vi "Update Humidity Control.vi"(8 "error in":errorcluster, 11 "cCRDS in":refnum<class "cCRDS.lvclass">=refnum) -> (0 "error out":errorcluster, 3 "cCRDS out":refnum<class "cCRDS.lvclass">)   [LabVIEW 2015, in "cCRDS.lvclass"]
uses:
  cCRDS.lvclass
  cCRDS.lvclass/cCRDS.ctl
  Reusable/CRDS/Cell/CRDS Cell.lvclass/CRDS Cell.ctl
  <vilib>/DAQmx/write.llb/DAQmx Write (Analog 1D DBL NChan 1Samp).vi
  Reusable/CRDS/Cell/Read Data.vi
  <vilib>/DAQmx/miscellaneous.llb/DAQmx Fill In Error Info.vi
  Reusable/CRDS/Main/Read Cells.vi
  Reusable/CRDS/Data/Cell/Read hkParam.vi
  Reusable/Humidity Control/Multi-Loop Humidity Control.vi
  Reusable/CRDS/Cell/CRDS Cell.lvclass
  Reusable/CRDS/Data/Cell/CRDS Cell Data.lvclass
  Reusable/General/Temperature/Temperature.lvlib
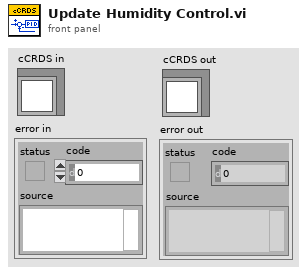
[diagram p1: front panel]
types:
  T1 = cluster{"Array of Single[0]":sgl, "Array of Single[1]":sgl, "Array of Single[2]":sgl}
  T2 = cluster{"Array of Single[0]":sgl, "Array of Single[1]":sgl, "Array of Single[2]":sgl}[]
  T3 = typedef "calData.ctl" = cluster{"rhDilFac":sgl, "Q":sgl, "Tmean":sgl, "extDilFac":sgl, "rhCell":sgl, "P":sgl, "T":sgl}
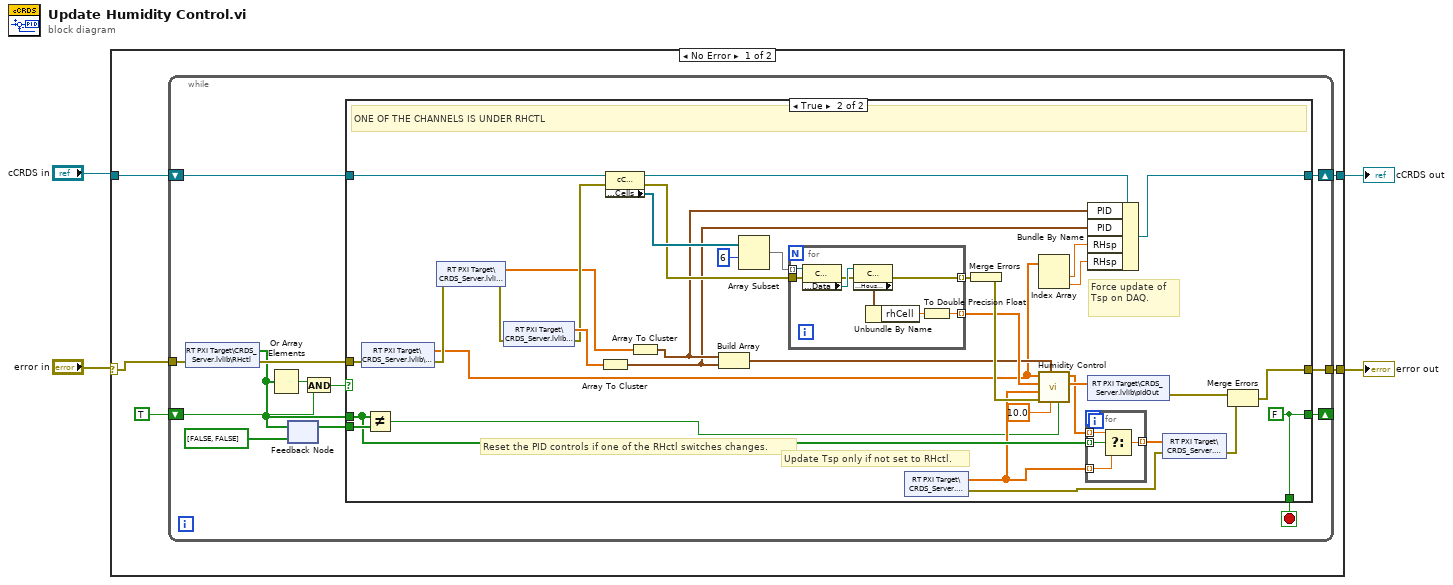
[diagram p0: block diagram]
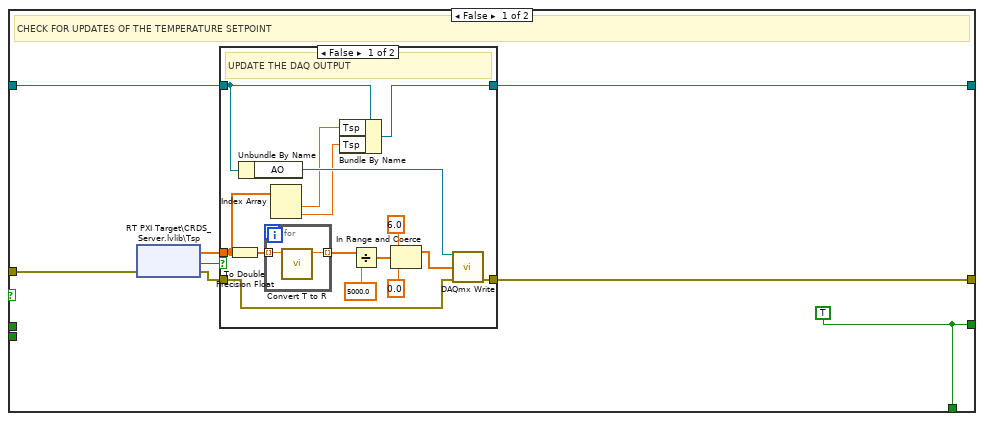
[diagram p2: hidden frame]
diagram:
  n1 = case shown="No Error" "error in" {
    selector: "error in" -> [w8 w98]
    tunnel: [w9 w98] -> w3
    tunnel: [w5 w97] -> w1
    tunnel: "cCRDS in" -> [w6 w97]
    frame No Error {
      n2 = while {
        tunnel: [w22] -> w9
        tunnel: w8 -> [w20]
        shift-right: [w18] -> _
        shift-left: TRUE -> [w17]
        shift-right: [w15] -> w5
        shift-left: w6 -> [w14]
        stop <- w19 stop-if-true
        n3 = shared-variable "RT PXI Target\\CRDS_Server.lvlib\\RHctl"(error in=w20) -> (w10:bool[], error out=w21:errorcluster)
        n4 = Or Array Elements(Boolean array=w10) -> (logical OR=w13:bool)
        n5 = feedback-in #1(w10) -> ()
        n6 = feedback #1(bool[] [FALSE, FALSE] ("Array of Boolean")) -> (w11:bool[])
        n7 = And(x=w13, y=w17) -> (x .and. y?=w16:bool)
        n8 = case shown="True" w16 {
          tunnel: [w30 w62] -> w22
          tunnel: w21 -> [w27 w77]
          tunnel: [w25 w72] -> w19
          tunnel: [w25 w72] -> w18
          tunnel: [w23 w65] -> w15
          tunnel: w14 -> [w24 w64]
          tunnel: w11 -> [_ w61]
          tunnel: w10 -> [_ w59]
          frame False {
            w25 = TRUE
            # "CHECK FOR UPDATES OF THE TEMPERATURE SETPOINT"
            n9 = shared-variable "RT PXI Target\\CRDS_Server.lvlib\\Tsp"(error in=w27) -> (w29:sgl[], error out=w26:errorcluster, w28:bool)  [unwired: 1 in]
            n10 = case shown="False" w28 {
              tunnel: w29 -> [w34 _]
              tunnel: [w44 w49] -> w30
              tunnel: w24 -> [w35 w48]
              tunnel: w26 -> [w41 w49]
              tunnel: [w31 w48] -> w23
              frame False {
                # "UPDATE THE DAQ OUTPUT"
                n11 = To Double Precision Float(number=w34) -> (double precision float=w36:dbl[])
                n12 = Unbundle By Name(w35) -> ("AO"=w45:refnum<k21>)
                n13 = for {
                  tunnel: w36 -> [w47] mode=indexing
                  tunnel: [w46] -> w42 mode=indexing
                  n14 = call "Convert T to R.vi"("T"=w47) -> ("R"=w46:dbl)  [unwired: 10 in]
                }
                n15 = Index Array(array=w34) -> (element #1=w33:sgl, element #2=w32:sgl)  [unwired: 2 in]
                n16 = Bundle By Name(cluster=w35, "Tsp"=w33, "Tsp"=w32) -> (w31:refnum<class "cCRDS.lvclass">)
                n17 = Divide(x=w42, y=5000.0) -> (x/y=w40:dbl[])
                n18 = In Range and Coerce(upper limit=6.0, x=w40, lower limit=0.0) -> (coerced(x)=w37:dbl[])  [unwired: 1 out]
                n19 = call-poly <vilib>:"DAQmx Write.vi"("task/channels in"=w45, "data"=w37, "error in"=w41) -> ("error out"=w44:errorcluster)  [unwired: 10 in, 2 out]
              }
              frame True {
                # "NO UPDATE"
              }
            }
          }
          frame True {
            w72 = FALSE
            # "Reset the PID controls if one of the RHctl switches changes."
            # "Update Tsp only if not set to RHctl."
            # "Force update of Tsp on DAQ."
            # "ONE OF THE CHANNELS IS UNDER RHCTL"
            n20 = shared-variable "RT PXI Target\\CRDS_Server.lvlib\\RHsp"(error in=w77) -> (w53:sgl[], error out=w76:errorcluster)
            n21 = Not Equal?(x=w59, y=w61) -> (x != y?=w50:bool)
            n22 = shared-variable "RT PXI Target\\CRDS_Server.lvlib\\Med"(error in=w76) -> (w70:sgl[], error out=w80:errorcluster)
            n23 = shared-variable "RT PXI Target\\CRDS_Server.lvlib\\High"(error in=w80) -> (w81:sgl[], error out=w78:errorcluster)
            n24 = Array To Cluster(array=w81) -> (cluster=w68:T1)
            n25 = property class="cCRDS"(reference=w64, error in=w78) -> (reference out=w71:refnum<class "cCRDS.lvclass">, error out=w79:errorcluster, "Data Access:Cells"=w84:refnum<class "CRDS Cell.lvclass">[])
            n26 = Array To Cluster(array=w70) -> (cluster=w69:T1)
            n27 = Build Array(w69, w68) -> (w54:T2)
            n28 = Array Subset(array=w84, index=6) -> (w82:refnum<class "CRDS Cell.lvclass">[])  [unwired: 1 in]
            n29 = for {
              tunnel: w82 -> [w96] mode=indexing
              tunnel: w79 -> [w92]
              tunnel: [w90] -> w75 mode=indexing
              tunnel: [w89] -> w73 mode=indexing
              n30 = property class="CRDS Cell"(reference=w96, error in=w92) -> (error out=w91:errorcluster, "Data Access:Data"=w95:refnum<class "CRDS Cell Data.lvclass">)  [unwired: 1 out]
              n31 = property class="CRDS Cell"(reference=w95, error in=w91) -> (error out=w90:errorcluster, "Data Access:Housekeeping"=w94:T3)  [unwired: 1 out]
              n32 = Unbundle By Name(w94) -> ("rhCell"=w93:sgl)
              n33 = To Double Precision Float(number=w93) -> (double precision float=w89:dbl)
            }
            n34 = shared-variable "RT PXI Target\\CRDS_Server.lvlib\\Tsp"() -> (w52:sgl[], error out=w55:errorcluster)  [unwired: 1 in]
            n35 = Merge Errors(w75) -> (w74:errorcluster)
            n36 = Index Array(array=w53) -> (element #1=w67:sgl, element #2=w66:sgl)  [unwired: 2 in]
            n37 = call-poly "Humidity Control.vi"("Reset?"=w50, "dt (s)"=10.0, "PID"=w54, "error in"=w74, "TspIn"=w52, "RH meas"=w73, "RHsp"=w53) -> ("PID Out"=w63:sgl[], "TspOut"=w60:sgl[])  [unwired: 2 in, 1 out]
            n38 = for {
              tunnel: w60 -> [w85] mode=indexing
              tunnel: w59 -> [w88] mode=indexing
              tunnel: w52 -> [w87] mode=indexing
              tunnel: [w86] -> w58 mode=indexing
              n39 = Select(t=w85, s=w88, f=w87) -> (s? t:f=w86:sgl)
            }
            n40 = Bundle By Name(cluster=w71, "PID"=w69, "PID"=w68, "RHsp"=w67, "RHsp"=w66) -> (w65:refnum<class "cCRDS.lvclass">)
            n41 = shared-variable "RT PXI Target\\CRDS_Server.lvlib\\pidOut"(w63) -> (error out=w56:errorcluster)  [unwired: 1 in]
            n42 = shared-variable "RT PXI Target\\CRDS_Server.lvlib\\Tsp"(w58, error in=w55) -> (error out=w57:errorcluster)
            n43 = Merge Errors(w56, w57) -> (w62:errorcluster)
          }
        }
      }
    }
    frame Error {
    }
  }
  "error out" <- w3
  "cCRDS out" <- w1
